vi "Get Test Case.vi"(7 "Start Time":timestamp, 10 "Assert Event Data":T3={"name"="", "passed"=FALSE, "call-chain"=[], "test-error"={"status"=FALSE, "code"=0, "source"=""}, "timestamp"=timestamp(0 s since 1904-01-01), "assert-id"="", "test-id"="", "time"=-1.0, "message"="", "properties"=variant, "measurements"=variant, "user-defined"=variant}) -> (2 "Test Case":T1)   [LabVIEW 2013, in "JUnit for Azure Pipelines.lvclass"]
uses:
  JUnit for Azure Pipelines.lvclass
  <vilib>/addons/_JKI Toolkits/Caraya/classes/Test Result/Assert Event Data (Extended).ctl
  Test Case.ctl
  Test Result.ctl
  <vilib>/addons/_JKI Toolkits/Caraya/classes/Test Result/Test Result.lvclass
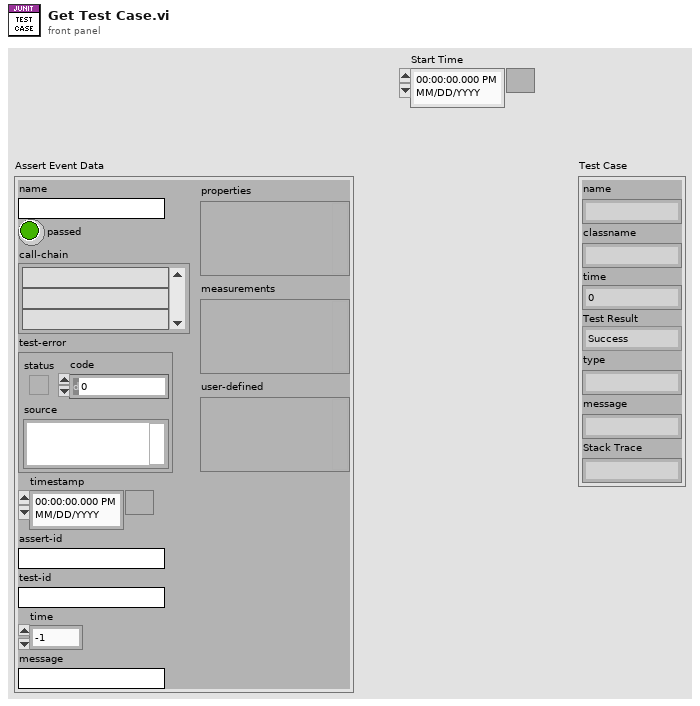
[diagram p1: front panel]
types:
  T1 = typedef "JUnit for Azure Pipelines.lvclass/Test Case.ctl" = cluster{"name":string, "classname":string, "time":dbl, "Test Result":T2, "type":string, "message":string, "Stack Trace":string}
  T2 = typedef "JUnit for Azure Pipelines.lvclass/Test Result.ctl" = enum16{"Success", "Failure", "Error", "Skipped"}
  T3 = typedef "Caraya.lvlib/Test Result.lvclass/Assert Event Data (Extended).ctl" = cluster{"name":string, "passed":bool, "call-chain":string[], "test-error":errorcluster, "timestamp":timestamp, "assert-id":string, "test-id":string, "time":dbl, "message":string, "properties":variant, "measurements":variant, "user-defined":variant}
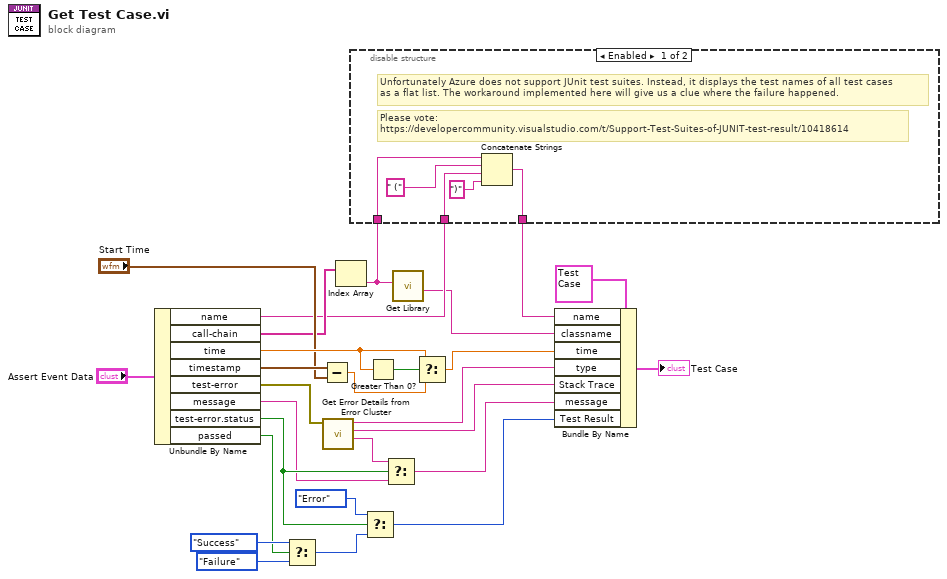
[diagram p0: block diagram]
diagram:
  n1 = Unbundle By Name("Assert Event Data") -> ("name"=w4:string, "call-chain"=w5:string[], "time"=w17:dbl, "timestamp"=w8:timestamp, "test-error"=w10:errorcluster, "message"=w14:string, "test-error.status"=w15:bool, "passed"=w20:bool)
  n2 = Select(t=Test_Result."Success" ("Test Result"), s=w20, f=Test_Result."Failure" ("Test Result")) -> (s? t:f=w23:T2)
  n3 = Subtract(x=w8, y="Start Time") -> (x-y=w7:dbl)
  n4 = call "Get Error Details from Error Cluster.vi"("error"=w10) -> ("Message"=w12:string, "Call Chain"=w13:string, "Source"=w9:string)  [unwired: 8 in]
  n5 = Index Array(array=w5) -> (element=w1:string)  [unwired: 1 in]
  n6 = disable-structure shown="Enabled" {
    disable-tunnel: w4 -> [w32 w33]
    disable-tunnel: [w30 w33] -> w3
    disable-tunnel: w1 -> [w31 _]
    frame Enabled {
      # "Unfortunately Azure does not support JUnit test suites. Instead, it displays the test names of all test cases\nas a flat list. The workaround implemented here will give us a clue where the failure happened."
      # "Please vote:\nhttps://developercommunity.visualstudio.com/t/Support-Test-Suites-of-JUNIT-test-result/10418614"
      n7 = Concatenate Strings(w31, " (" ("string"), w32, ")" ("string")) -> (w30:string)
    }
    frame Disabled {
    }
  }
  n8 = Select(t=Test_Result."Error" ("Test Result"), s=w15, f=w23) -> (s? t:f=w19:T2)
  n9 = Greater Than 0?(x=w17) -> (x > 0?=w18:bool)
  n10 = Select(t=w12, s=w15, f=w14) -> (s? t:f=w11:string)
  n11 = call "Get Library.vi"("Call Chain"=w1) -> ("Name"=w2:string)  [unwired: 9 in, 1 out]
  n12 = Select(t=w17, s=w18, f=w7) -> (s? t:f=w16:dbl)
  n13 = Bundle By Name(cluster=T1 {"name"="", "classname"="", "time"=0.0, "Test Result"=enum."Success", "type"="", "message"="", "Stack Trace"=""} ("Test Case"), "name"=w3, "classname"=w2, "time"=w16, "type"=w9, "Stack Trace"=w13, "message"=w11, "Test Result"=w19) -> (→"Test Case":T1)
